vi "DriveAtAngle.vi"(0 "Target Angle":dbl, 1 "Distance":dbl, 3 "Error In":errorcluster) -> (7 "y-axis distance":dbl, 8 "x":dbl, 9 "y":dbl, 10 "Error Out":errorcluster)   [LabVIEW 2017]
panel:
  out "x power":dbl
  out "y power":dbl
  # "DriveAtAngle Autonomous Commands\nTeam 34 Rockets"
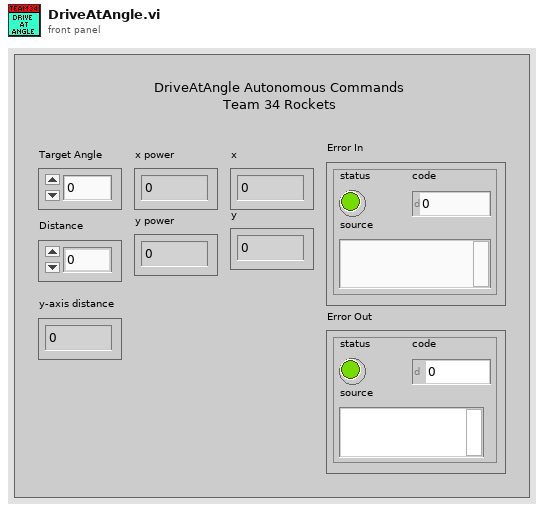
[diagram p1: front panel]
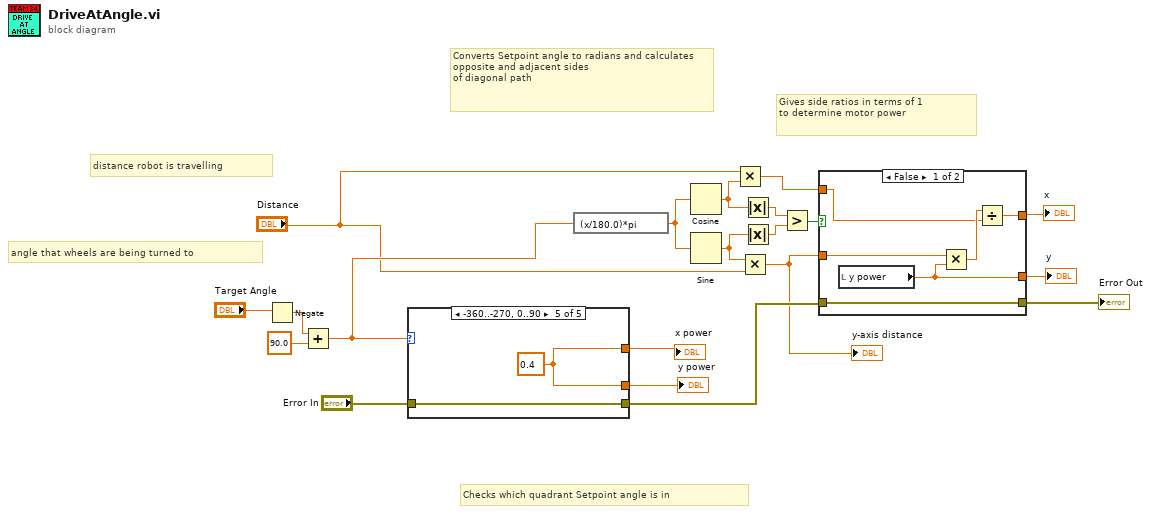
[diagram p0: block diagram]
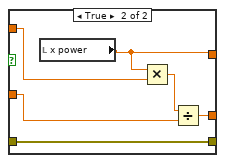
[diagram p2: hidden frame]
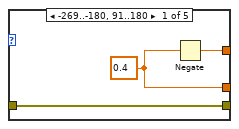
[diagram p3: hidden frame]
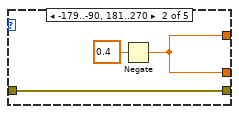
[diagram p4: hidden frame]
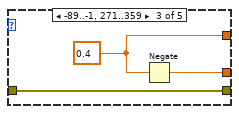
[diagram p5: hidden frame]
diagram:
  # "Checks which quadrant Setpoint angle is in"
  # "Gives side ratios in terms of 1\nto determine motor power"
  # "Converts Setpoint angle to radians and calculates opposite and adjacent sides \nof diagonal path"
  # "distance robot is travelling"
  # "angle that wheels are being turned to"
  n1 = Negate(x="Target Angle") -> (-x=w18:dbl)
  n2 = Add(x=w18, y=90.0) -> (x+y=w17:dbl)
  n3 = case shown="-360..-270, 0..90" w17 {
    tunnel: [w21 w25 w28 _ w31] -> w4
    tunnel: [w22 w25 w27 _ w31] -> w3
    tunnel: "Error In" -> [w23 w26 w29 w30 w32]
    tunnel: [w23 w26 w29 w30 w32] -> w9
    frame -269..-180, 91..180 {
      w21 = 0.4
      n4 = Negate(x=w21) -> (-x=w22:dbl)
    }
    frame -179..-90, 181..270 {
      n5 = Negate(x=0.4) -> (-x=w25:dbl)
    }
    frame -89..-1, 271..359 {
      w27 = 0.4
      n6 = Negate(x=w27) -> (-x=w28:dbl)
    }
    frame Default {
    }
    frame -360..-270, 0..90 {
      w31 = 0.4
    }
  }
  "x power" <- w3
  "y power" <- w4
  n7 = expression code="(x/180.0)*pi"(w17) -> (w20:dbl)
  n8 = Cosine(x=w20) -> (cos(x)=w14:dbl)
  n9 = Sine(x=w20) -> (sin(x)=w13:dbl)
  n10 = Multiply(x="Distance", y=w14) -> (x*y=w15:dbl)
  n11 = Multiply(x=w13, y="Distance") -> (x*y=w2:dbl)
  "y-axis distance" <- w2
  n12 = Absolute Value(x=w14) -> (abs(x)=w11:dbl)
  n13 = Absolute Value(x=w13) -> (abs(x)=w12:dbl)
  n14 = Greater?(x=w11, y=w12) -> (0:w8:bool)
  n15 = case shown="False" w8 {
    tunnel: [w33 w43] -> w7
    tunnel: [w38 w39] -> w6
    tunnel: w2 -> [w36 w42]
    tunnel: w15 -> [w35 w41]
    tunnel: w9 -> [w34 w40]
    tunnel: [w34 w40] -> w5
    frame False {
      n16 = local read "y power"() -> (w33:dbl)
      n17 = Multiply(x=w36, y=w33) -> (x*y=w37:dbl)
      n18 = Divide(x=w37, y=w35) -> (x/y=w38:dbl)
    }
    frame True {
      n19 = local read "x power"() -> (w39:dbl)
      n20 = Multiply(x=w39, y=w41) -> (x*y=w44:dbl)
      n21 = Divide(x=w44, y=w42) -> (x/y=w43:dbl)
    }
  }
  "Error Out" <- w5
  "x" <- w6
  "y" <- w7
